vi "数据补发判定有限循环.vi"(8 "错误输入（无错误）":errorcluster, 9 "数据输入":string, 11 "数据发送通道":enum16{"TCP", "VISA"}(ring)) -> (3 "error out":errorcluster)   [LabVIEW 2016, in "数据传输系统.lvlib"]
uses:
  <vilib>/ptbypt/NI_PtbyPt.lvlib
panel:
  out "重发次数":dbl
  out "x+1":u32
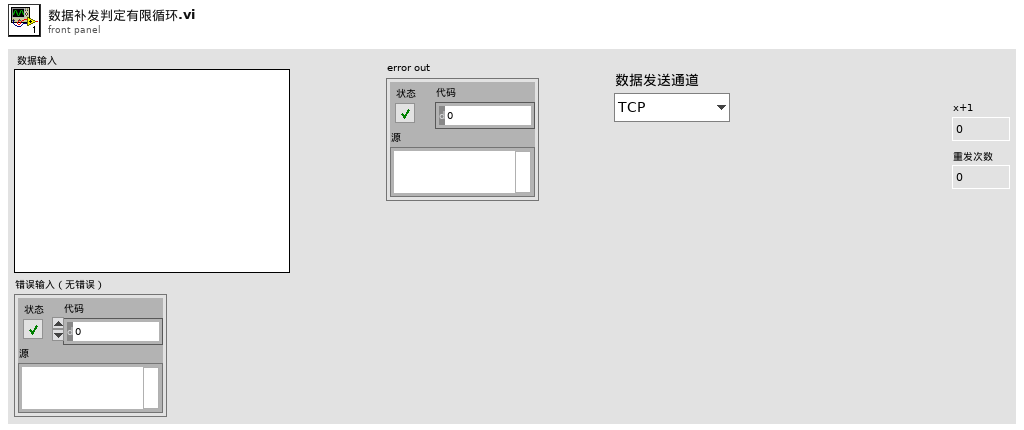
[diagram p1: front panel]
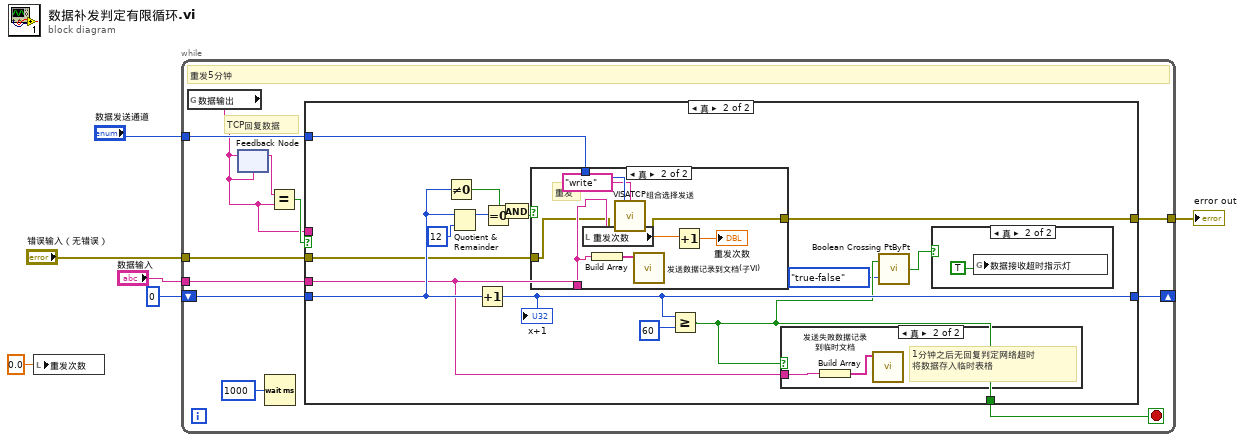
[diagram p0: block diagram]
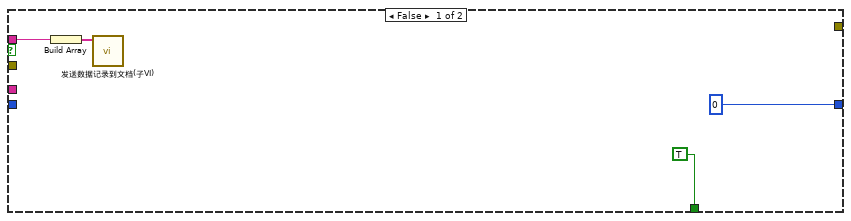
[diagram p2: hidden frame]
diagram:
  n1 = local write "重发次数"(0.0 ("重发次数")) -> ()
  n2 = while {
    shift-right: [w15] -> _
    shift-left: u32 0 ("等待时间（毫秒）") -> [w16]
    tunnel: "数据发送通道" -> [w11]
    tunnel: [w10] -> w5
    tunnel: "数据输入" -> [w9]
    tunnel: "错误输入（无错误）" -> [w8]
    stop <- w14 stop-if-true
    # "TCP回复数据"
    # "重发5分钟"
    n3 = global read "全局1.vi" "数据输出"() -> (w7:string)
    n4 = feedback-in #1(w7) -> ()
    n5 = feedback #1(w7) -> (w13:string)
    n6 = Wait (ms)(milliseconds to wait=u32 1000 ("等待时间（毫秒）")) -> ()  [unwired: 1 out]
    n7 = Equal?(x=w13, y=w7) -> (x = y?=w12:bool)
    n8 = case shown="真" w12 {
      tunnel: w16 -> [_ w30]
      tunnel: [u32 0 w35] -> w15
      tunnel: [TRUE w24] -> w14
      tunnel: w11 -> [_ w28]
      tunnel: [_ w27] -> w10
      tunnel: w9 -> [_ w25]
      tunnel: w8 -> [_ w26]
      tunnel: w7 -> [w18 _]
      frame False {
        n9 = Build Array(w18) -> (w19:string[])
        n10 = call "发送数据记录到文档(子VI).vi"("数组"=w19) -> ()  [unwired: 9 in, 1 out]
      }
      frame True {
        n11 = Not Equal To 0?(x=w30) -> (x != 0?=w29:bool)
        n12 = Quotient & Remainder(x=w30, y=u32 12) -> (x-y*floor(x/y)=w33:u32)  [unwired: 1 out]
        n13 = Increment(x=w30) -> (x+1=w35:u32)
        "x+1" <- w35
        n14 = Equal To 0?(x=w33) -> (x = 0?=w32:bool)
        n15 = And(x=w29, y=w32) -> (x .and. y?=w31:bool)
        n16 = case shown="真" w31 {
          tunnel: w28 -> [_ w45]
          tunnel: [w40 w41] -> w27
          tunnel: w25 -> [_ w43]
          tunnel: w26 -> [w40 w42]
          frame False {
          }
          frame True {
            # "重发"
            n17 = local read "重发次数"() -> (w47:dbl)
            n18 = Build Array(w43) -> (w46:string[])
            n19 = call "VISATCP组合选择发送.vi"("数据发送通道"=w45, "命令"="write", "error in (no error)"=w42, "写入缓冲区"=w43) -> ("错误输出"=w41:errorcluster)  [unwired: 8 in, 3 out]
            n20 = call "发送数据记录到文档(子VI).vi"("数组"=w46) -> ()  [unwired: 9 in, 1 out]
            n21 = Increment(x=w47) -> (x+1=→"重发次数":dbl)
          }
        }
        n22 = Greater Or Equal?(x=w35, y=u32 60) -> (x >= y?=w24:bool)
        n23 = case shown="真" w24 {
          tunnel: w25 -> [_ w38]
          frame False {
          }
          frame True {
            # "1分钟之后无回复判定网络超时\n将数据存入临时表格"
            n24 = Build Array(w38) -> (w39:string[])
            n25 = call "发送失败数据记录到临时文档.vi"("数组"=w39) -> ()  [unwired: 9 in, 1 out]
          }
        }
        n26 = call <vilib>:"Boolean Crossing PtByPt.vi"("direction"=enum16{"either", "false-true", "true-false"}."true-false", "input"=w24) -> ("crossing"=w22:bool)  [unwired: 1 in]
        n27 = case shown="真" w22 {
          frame False {
          }
          frame True {
            n28 = global write "全局 数据发送重叠.vi" "数据接收超时指示灯"(TRUE ("数据接收超时指示灯")) -> ()
          }
        }
      }
    }
  }
  "error out" <- w5
